vi "lockin.SMO.vi"() -> ()   [LabVIEW 2016]
uses:
  <vilib>/JKI/JKI SMO/SMO/Typedefs/SMOState --Enum.ctl
  SMOs/DAQ/Typedefs/DAQ.Config.ctl
  SMOs/DAQ/Typedefs/PrivateEvents--DAQ.AI.Channels.ctl
  SMOs/DAQ/Typedefs/DAQType.ctl
  SMOs/DAQ/Typedefs/SamplingInfo.ctl
  SMOs/DAQ/Typedefs/SamplingMode.ctl
  SMOs/DAQmx.AI/Typedefs/DAQmx.AI.Config.ctl
  SMOs/DAQmx.AO/Typedefs/DAQmx.AO.Config.ctl
  SMOs/DAQmx/DAQmx.lvclass
  C:/user/patrick/hg/lockin.SMO/lvsrc/SMOs/DAQ/DAQ.lvclass
  SMOs/DAQmx.AI/DAQmx.AI.lvclass
  C:/user/patrick/hg/lockin.SMO/lvsrc/SMOs/DAQmx/DAQmx.lvclass
  SMOs/DAQmx.AO/DAQmx.AO.lvclass
  SMOs/DAQ/DAQ.lvclass
  C:/Program Files (x86)/National Instruments/LabVIEW 2016/vi.lib/JKI/JKI SMO/SMO/SMO.lvclass
  <vilib>/JKI/JKI SMO/SMO/SMO.lvclass
panel:
  in  "DAQmx.AO.config":T1={"output terminal configuration"=-1} {"output terminal configuration" items=["Default"=-1, "RSE"=10083, "Differential"=10106, "Pseudodifferential"=12529]}
  in  "DAQmx.AI.config":T2={"AI.Coupling"=10045, "input terminal configuration "=-1} {"input terminal configuration" items=["default"=-1, "RSE"=10083, "NRSE"=10078, "Differential"=10106, "Pseudodifferential"=12529]; "AI.Coupling" items=["AC"=10045, "DC"=10050, "GND"=10066]}
  in  "DAQmx Physical Channel":tag
  in  "DAQ.Config":T3={"Channels"="", "DAQType"=enum."AI", "minimum value"=-5.0, "maximum value"=5.0, "sampling info"={"Fs"=1000.0, "#s"=1000.0}, "SamplingMode"=enum."Continuous"} {"maximum value" format="%0.2f"; "minimum value" format="%0.2f"}
  in  "Simulate?":bool
  out "Write":T8(graph)
  out "Read":T9(graph)
  out "SMO State":T10
  out "error out":errorcluster
  in  "Stop":bool
  # "Lockin SMO Test Launcher"
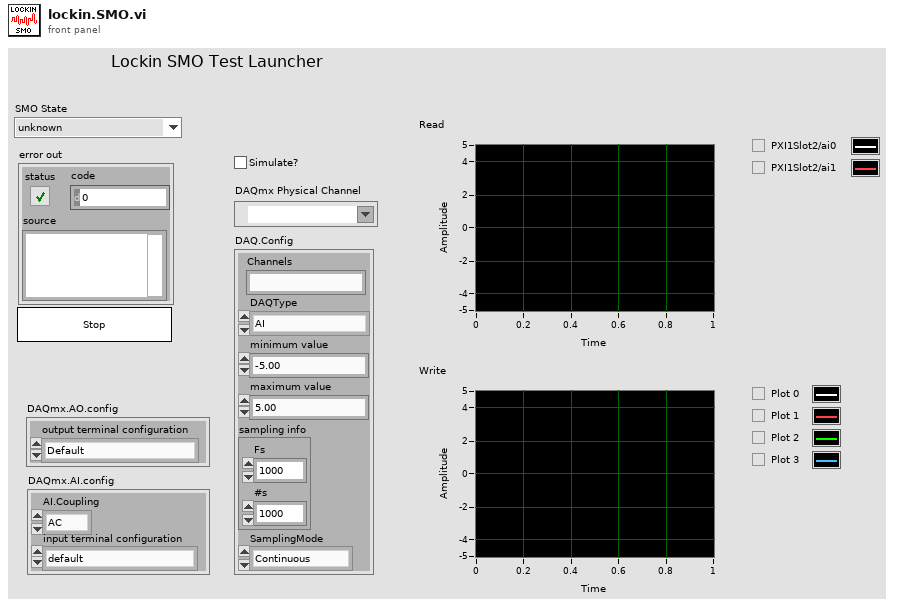
[diagram p1: front panel]
types:
  T1 = typedef "DAQmx.AO.lvclass/DAQmx.AO.Config.ctl" = cluster{"output terminal configuration":i32}
  T2 = typedef "DAQmx.AI.lvclass/DAQmx.AI.Config.ctl" = cluster{"AI.Coupling":i32, "input terminal configuration ":i32}
  T3 = typedef "DAQ.lvclass/DAQ.Config.ctl" = cluster{"Channels":T4, "DAQType":T5, "minimum value":dbl, "maximum value":dbl, "sampling info":T6, "SamplingMode":T7}
  T4 = typedef "DAQ.lvclass/PrivateEvents--DAQ.AI.Channels.ctl" = string
  T5 = typedef "DAQ.lvclass/DAQType.ctl" = enum16{"AI", "AO"}
  T6 = typedef "DAQ.lvclass/SamplingInfo.ctl" = cluster{"Fs":dbl, "#s":dbl}
  T7 = typedef "DAQ.lvclass/SamplingMode.ctl" = enum16{"Continuous", "Finite"}
  T8 = typedef "DAQ.lvclass/PublicEvents--DAQ.Write.ctl" = waveform(dbl)[]
  T9 = typedef "DAQ.lvclass/PublicEvents--DAQ.Read.ctl" = waveform(dbl)[]
  T10 = typedef "SMO.lvclass/SMOState --Enum.ctl" = enum16{"unknown", "Created", "Started", "Stopped"}
  T11 = typedef "SMO.lvclass/Public Events.ctl" = cluster{"Error":refnum<user-event>, "State":refnum<user-event>, "Reserve State":refnum<user-event>}
  T12 = typedef "DAQ.lvclass/PublicEvents--Cluster.ctl" = cluster{"Read":refnum<user-event>, "Write":refnum<user-event>}
  T13 = cluster{"Event Registration Refnum":refnum<event-registration>}
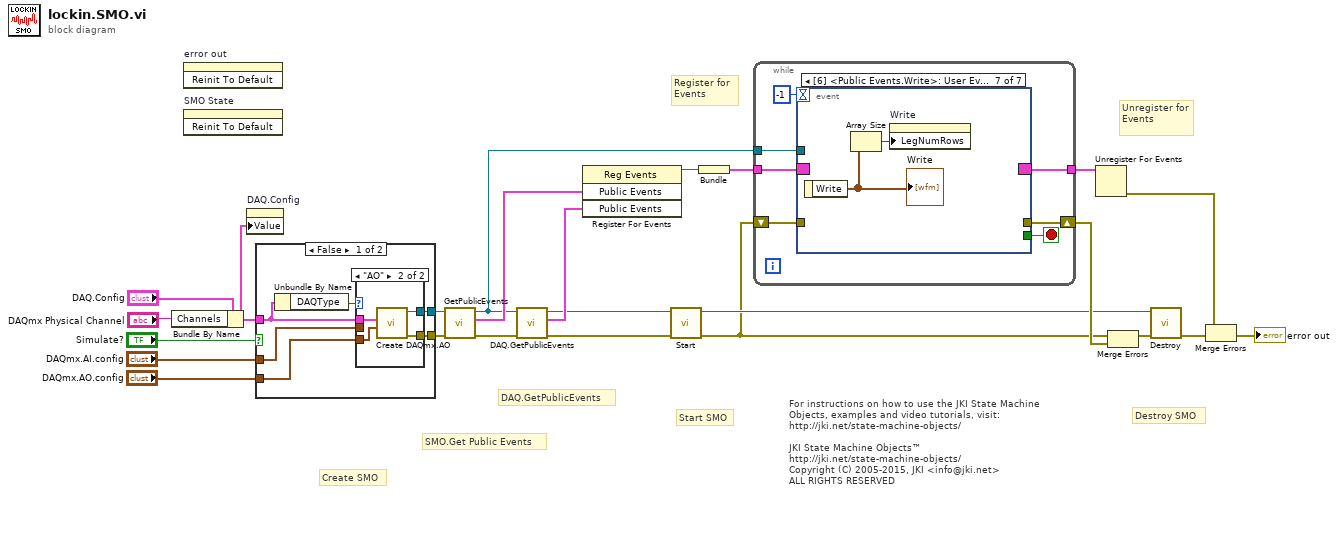
[diagram p0: block diagram]
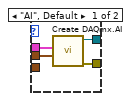
[diagram p2: hidden frame]
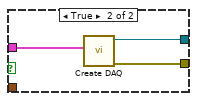
[diagram p3: hidden frame]
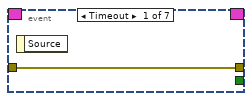
[diagram p4: hidden frame]
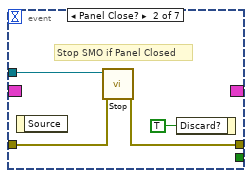
[diagram p5: hidden frame]
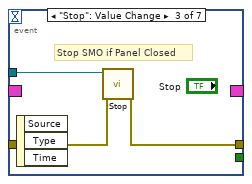
[diagram p6: hidden frame]
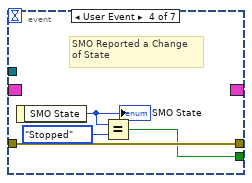
[diagram p7: hidden frame]
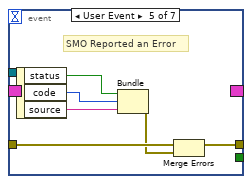
[diagram p8: hidden frame]
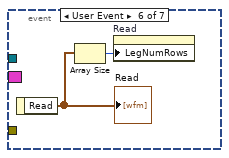
[diagram p9: hidden frame]
diagram:
  # "DAQ.GetPublicEvents"
  # "For instructions on how to use the JKI State Machine Objects, examples and video tutorials, visit:\nhttp://jki.net/state-machine-objects/\n\nJKI State Machine Objects™\nhttp://jki.net/state-machine-objects/\nCopyright (C) 2005-2015, JKI <info@jki.net>\nALL RIGHTS RESERVED"
  # "SMO.Get Public Events"
  # "Start SMO"
  # "Destroy SMO"
  # "Create SMO"
  # "Unregister for Events"
  # "Register for Events"
  n1 = Bundle By Name(cluster="DAQ.Config", "Channels"="DAQmx Physical Channel") -> (w1:T3)
  n2 = invoke on="error out" class="Clust (strict)" method="Reinit To Default"() -> ()  [unwired: 3 in, 3 out]
  n3 = invoke on="SMO State" class="Enum (strict)" method="Reinit To Default"() -> ()  [unwired: 3 in, 3 out]
  n4 = property on="DAQ.Config" class="Clust (strict)"("Value"=w1) -> ()  [unwired: 2 in, 2 out]
  n5 = case shown="False" "Simulate?" {
    tunnel: w1 -> [w29 w41]
    tunnel: [w27 w40] -> w5
    tunnel: [w28 w39] -> w4
    tunnel: "DAQmx.AI.config" -> [w26 _]
    tunnel: "DAQmx.AO.config" -> [w25 _]
    frame False {
      n6 = Unbundle By Name(w29) -> ("DAQType"=w30:T5)
      n7 = case shown="\"AO\"" w30 {
        tunnel: w29 -> [w34 w38]
        tunnel: [w32 w37] -> w28
        tunnel: [w33 w36] -> w27
        tunnel: w26 -> [w31 _]
        tunnel: w25 -> [_ w35]
        frame "AI", Default {
          n8 = call "Create DAQmx.AI.vi"("DAQmx.AI.config"=w31, "DAQ.config"=w34) -> ("error out"=w33:errorcluster, "DAQmx.AI out"=w32:refnum<class "DAQmx.AI.lvclass">)  [unwired: 8 in]
        }
        frame "AO" {
          n9 = call "Create DAQmx.AO.vi"("DAQmx.AO.config"=w35, "DAQ.Config"=w38) -> ("error out"=w36:errorcluster, "DAQmx.AO out"=w37:refnum<class "DAQmx.AO.lvclass">)  [unwired: 8 in]
        }
      }
    }
    frame True {
      n10 = call "Create DAQ.vi"("DAQ.Config"=w41) -> ("error out"=w40:errorcluster, "DAQ out"=w39:refnum<class "DAQ.lvclass">)  [unwired: 9 in]
    }
  }
  n11 = call <vilib>:"GetPublicEvents.vi"("error in (no error)"=w5, "SMO"=w4) -> ("error out"=w13:errorcluster, "Public Events"=w16:T11, "SMO out"=w14:refnum<class "DAQ.lvclass">)  [unwired: 7 in]
  n12 = call "DAQ.GetPublicEvents.vi"("error in (no error)"=w13, "DAQ"=w14) -> ("error out"=w8:errorcluster, "Public Events"=w12:T12, "DAQ out"=w9:refnum<class "DAQ.lvclass">)  [unwired: 7 in]
  n13 = register-events(w16, w12) -> (reference out=w15:refnum<event-registration>)  [unwired: 2 in, 1 out]
  n14 = call <vilib>:"Start.vi"("error in (no error)"=w8, "SMO"=w9) -> ("error out"=w11:errorcluster, "SMO out"=w17:refnum<class "DAQ.lvclass">)  [unwired: 8 in]
  n15 = Bundle("Event Registration Refnum"=w15) -> (w23:T13)  [unwired: 1 in]
  n16 = while {
    shift-right: [w47] -> w22
    shift-left: w11 -> [w46]
    tunnel: w23 -> [w45]
    tunnel: [w44] -> w24
    tunnel: w14 -> [w43]
    stop <- w48 stop-if-true
    n17 = event shown="[6] <Public Events.Write>: User Event" {
      selector: w45 -> [_ _ _ _ _ _ _]
      dyn-events: [_ _ _ _ _ _ _] -> w44
      timeout: -1 -> [_ _ _ _ _ _ _]
      tunnel: [_ _ _ w57 _ _ _] -> w48
      tunnel: w43 -> [_ w53 w56 _ _ _ _]
      tunnel: [w49 w52 w55 w60 w64 _ _] -> w47
      tunnel: w46 -> [w49 w51 w54 w60 w62 _ _]
      event Timeout {
        n18 = event-data() -> ()  [unwired: 1 in, 1 out]
      }
      event Panel Close? {
        # "Stop SMO if Panel Closed"
        n19 = event-data() -> ()  [unwired: 1 in, 1 out]
        n20 = call <vilib>:"Stop.vi"("error in (no error)"=w51, "SMO"=w53) -> ("error out"=w52:errorcluster)  [unwired: 8 in, 1 out]
        n21 = event-data("Discard?"=TRUE ("OK")) -> ()  [unwired: 1 in, 1 out]
      }
      event "Stop": Value Change {
        # "Stop SMO if Panel Closed"
        n22 = event-data() -> ()  [unwired: 1 in, 3 out]
        n23 = call <vilib>:"Stop.vi"("error in (no error)"=w54, "SMO"=w56) -> ("error out"=w55:errorcluster)  [unwired: 8 in, 1 out]
      }
      event User Event {
        # "SMO Reported a Change\nof State"
        n24 = event-data() -> ("SMO State"=w59:T10)  [unwired: 1 in]
        "SMO State" <- w59
        n25 = Equal?(x=w59, y=SMOState_--Enum."Stopped") -> (x = y?=w57:bool)
      }
      event User Event {
        # "SMO Reported an Error"
        n26 = event-data() -> ("status"=w63:bool, "code"=w66:i32, "source"=w65:string)  [unwired: 1 in]
        n27 = Bundle("status"=w63, "code"=w66, "source"=w65) -> (w61:errorcluster)  [unwired: 1 in]
        n28 = Merge Errors(w62, w61) -> (w64:errorcluster)
      }
      event User Event {
        n29 = event-data() -> ("Read"=w67:T9)  [unwired: 1 in]
        "Read" <- w67
        n30 = Array Size(array=w67) -> (size(s)=w68:i32)
        n31 = property on="Read" class="WFGraph (strict)"("LegNumRows"=w68) -> ()  [unwired: 2 in, 2 out]
      }
      event User Event {
        n32 = event-data() -> ("Write"=w69:T8)  [unwired: 1 in]
        "Write" <- w69
        n33 = Array Size(array=w69) -> (size(s)=w70:i32)
        n34 = property on="Write" class="WFGraph (strict)"("LegNumRows"=w70) -> ()  [unwired: 2 in, 2 out]
      }
    }
  }
  n35 = Unregister For Events(event registration refnum=w24) -> (error out=w21:errorcluster)  [unwired: 1 in]
  n36 = Merge Errors(w11, w22) -> (w18:errorcluster)
  n37 = call <vilib>:"Destroy.vi"("error in (no error)"=w18, "SMO"=w17) -> ("error out"=w19:errorcluster)  [unwired: 9 in]
  n38 = Merge Errors(w21, w19) -> (→"error out":errorcluster)
